vi "Create Recipe Controller.vi"(7 "2-Axis Stage Async API.lvclass":refnum<class "2-Axis Stage Async API.lvclass">, 8 "error in (no error)":errorcluster, 9 "DAQ API.lvclass":refnum<class "DAQ API.lvclass">, 10 "Camera Controller":refnum<class "Camera Controller.lvclass">, 11 "Laser API.lvclass":refnum<class "Laser API.lvclass">) -> (0 "error out":errorcluster, 3 "Recipe Controller.lvclass":refnum<class "Recipe Controller.lvclass">)   [LabVIEW 2022 SP3, in "Recipe Controller.lvclass"]
uses:
  Recipe Controller.lvclass
  Camera/Camera Controller/Camera Controller.lvclass
  Laser/Laser Controller api/Laser API.lvclass
  IO Monitor/DAQ API/DAQ API.lvclass
  XY Stage/Interfaces/2-Axis Stage API/2-Axis Stage Async API.lvclass
  Recipe Controller.lvclass/Recipe Controller.ctl
  Recipe Process/Recipe Process/Recipe Process.lvclass
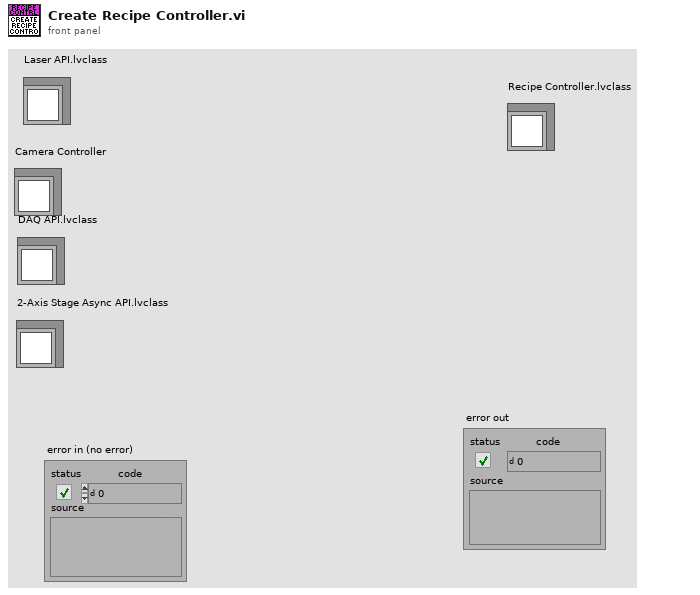
[diagram p1: front panel]
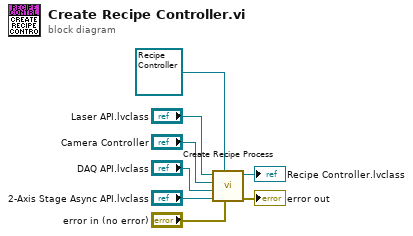
[diagram p0: block diagram]
diagram:
  n1 = call "Create Recipe Process.vi"("error in (no error)"="error in (no error)", "Recipe Controller.lvclass"=refnum<class "Recipe Controller.lvclass"> refnum, "2-Axis Stage Async API.lvclass"="2-Axis Stage Async API.lvclass", "DAQ API.lvclass"="DAQ API.lvclass", "Camera Controller"="Camera Controller", "Laser API.lvclass"="Laser API.lvclass") -> ("error out"=→"error out":errorcluster, "Recipe Controller.lvclass"=→"Recipe Controller.lvclass":refnum<class "Recipe Controller.lvclass">)  [unwired: 4 in]
